vi "LDA_Align_PN_8 point.vi"(1 "Align Probe Using":enum16{"Green Beams", "Blue Beams"}(ring), 2 "Use Specification Beam Half-Angle":bool) -> (0 "Beam Data":T2={"Vg1 (Green 1 dir. vect.)"=[0.059117350659853476, -0.996541267827751, 0.05840068807144843], "Vg2  (Green 2 dir. vect.)"=[-0.05232536310393669, -0.9971561380468801, -0.054237373935992664], "Vb1 (Blue 1 dir. vect.)"=[-0.052923229613528855, -0.9969242065933935, 0.057803616456121795], "Vb2 (Blue 1 dir. vect.)"=[0.05971521716944564, -0.9967731992812374, -0.05364030232066602], "Porb (Orb XYZ posn. forced coplanar)"=[2201.0738225655555, -1199.3737231995547, 269.758310600838], "Porb (Orb XYZ posn. - allow skew)"=[2200.796256301178, -1199.3740953152687, 270.0329332816893], "Orb posn. uncertainty, +/- dx, dy, dz"=[0.13878313218879157, 0.00018605785703584843, 0.13731134042564008], "Vp (Actual Probe dir. vect)"=[0.003406702197773746, -0.9999920168246164, 0.0020882210543692924], "Yaw (deg)"=89.80480953887573, "Pitch (deg)"=0.11964634006213794, "In-Plane Roll (deg)"=45.305328966424156, "Beam Half Angle (deg)"=4.544091484248422, "B1 Close P11"=[0.0, 0.0, 0.0], "B1 Far P12"=[2158.01, -491.04, 229.28], "B2 Close P22"=[2158.01, -491.04, 229.28], "B2 Far P21"=[2158.01, -491.04, 229.28], "Projected Roll (deg)"=0.0, "Green Velocity Vector"=[0.0, 0.0, 0.0], "Blue Velocity Vector"=[0.0, 0.0, 0.0], "Probe is facing...."="-", "Calculation Method"=""} {"Vp (Actual Probe dir. vect)" format="%#_6f"; "Vg2  (Green 2 dir. vect.)" format="%#_6f"; "Vg1 (Green 1 dir. vect.)" format="%#_6f"})   [LabVIEW 2018]
uses:
  Controls/LDA_Beam_Cluster.ctl
  Gen Trav/Route mapping/Axis.ctl
  Controls/Tunnel_Coordinates.ctl
  Controls/Post_Process.ctl
  Controls/Setup.ctl
  Controls/User_Specific_mode.ctl
  Globals/LDA_meas_global_1.vi
  Globals/Trav_pos_global.vi
panel:
  out "8 Peaked positions":dbl[][](array[numeric])
  out "Peakup up inputs":dbl[][](array[numeric])
  out "Fixed Axis":T1
  out "png folder":path
  out "Taught point names":string[](array[string])
  out "Taught Positions":dbl[][](array[numeric])
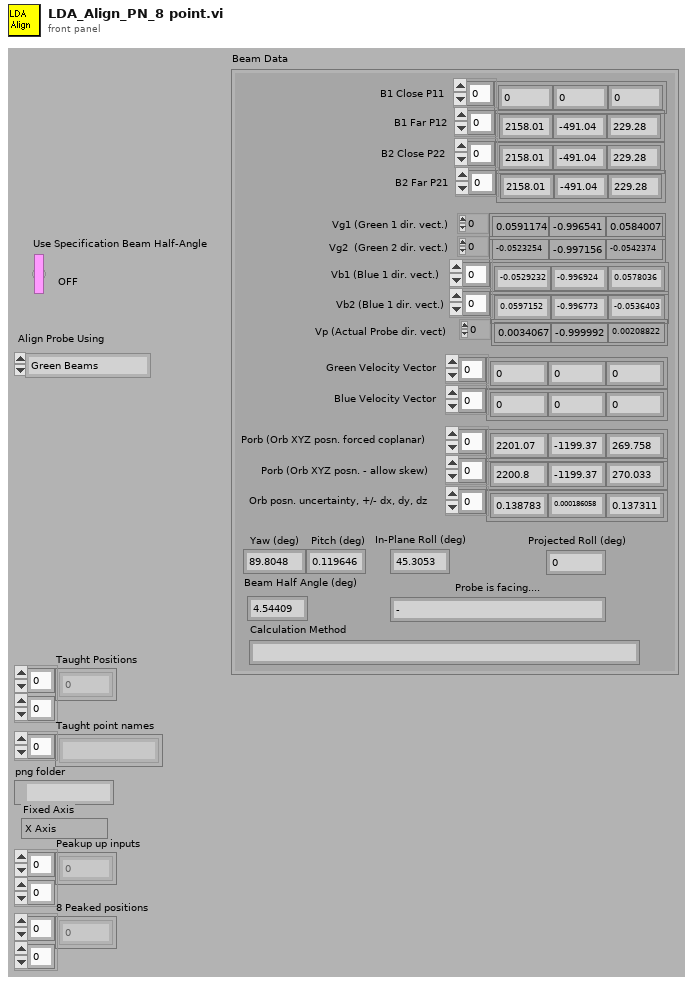
[diagram p1: front panel]
types:
  T1 = typedef "Axis.ctl" = enum16{"X Axis", "X Axis -ve", "Y Axis", "Y Axis -ve", "Z Axis", "Z Axis -ve"}
  T2 = typedef "LDA_Beam_Cluster.ctl" = cluster{"Vg1 (Green 1 dir. vect.)":dbl[], "Vg2  (Green 2 dir. vect.)":dbl[], "Vb1 (Blue 1 dir. vect.)":dbl[], "Vb2 (Blue 1 dir. vect.)":dbl[], "Porb (Orb XYZ posn. forced coplanar)":dbl[], "Porb (Orb XYZ posn. - allow skew)":dbl[], "Orb posn. uncertainty, +/- dx, dy, dz":dbl[], "Vp (Actual Probe dir. vect)":dbl[], "Yaw (deg)":dbl, "Pitch (deg)":dbl, "In-Plane Roll (deg)":dbl, "Beam Half Angle (deg)":dbl, "B1 Close P11":dbl[], "B1 Far P12":dbl[], "B2 Close P22":dbl[], "B2 Far P21":dbl[], "Projected Roll (deg)":dbl, "Green Velocity Vector":dbl[], "Blue Velocity Vector":dbl[], "Probe is facing....":string, "Calculation Method":string}
  T3 = typedef "Tunnel_Coordinates.ctl" = enum16{"Work in Tunnel Coordinates", "Work in Model Coordinates"}
  T4 = typedef "Setup.ctl" = enum16{"Run Program", "Show Setup", "Save Current Setup", "Setup Front Panel"}
  T5 = typedef "Post_Process.ctl" = enum16{"Take New Data", "Post Process Raw Data File"}
  T6 = typedef "User_Specific_mode.ctl" = enum16{"Check VI only", "Run VI"}
  T7 = enum16{"Load setup from excel file", "Save setup to excel file"}
  T8 = cluster{"second":i32, "minute":i32, "hour":i32, "day of month":i32, "month":i32, "year":i32, "day of week":i32, "day of year":i32, "is DST":i32}
  T9 = typedef "Multi_Run_Status.ctl" = enum16{"Continue", "Continue with Error", "Jump to Next Point", "Jump to Next Row", "Jump To Fall Back", "Terminate Run"}
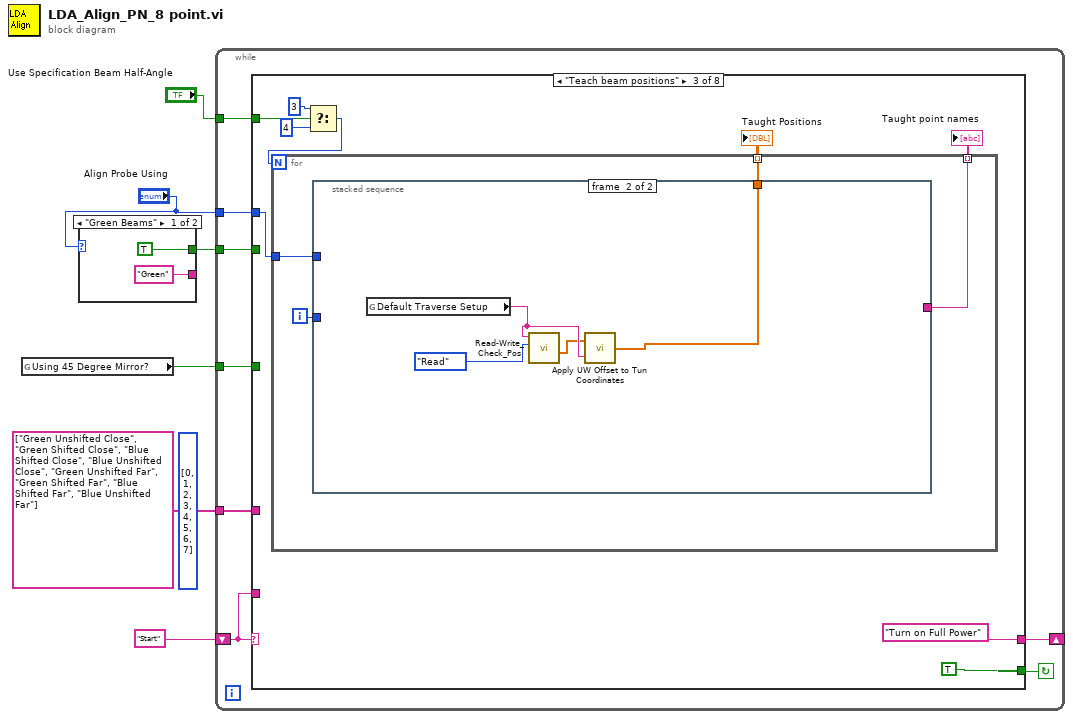
[diagram p0: block diagram]
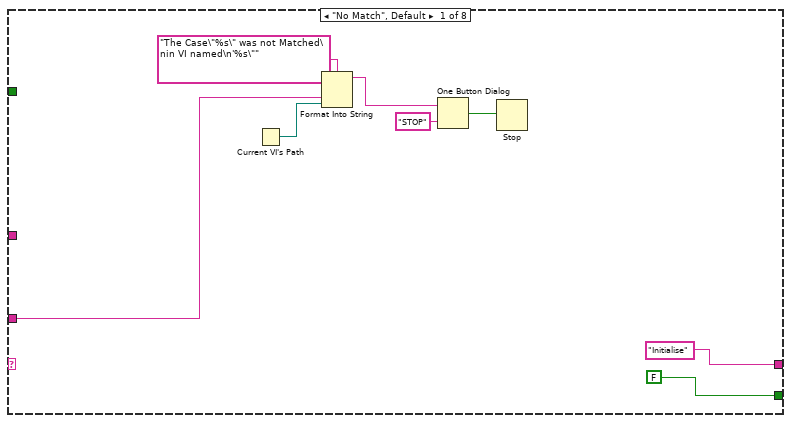
[diagram p2: hidden frame]
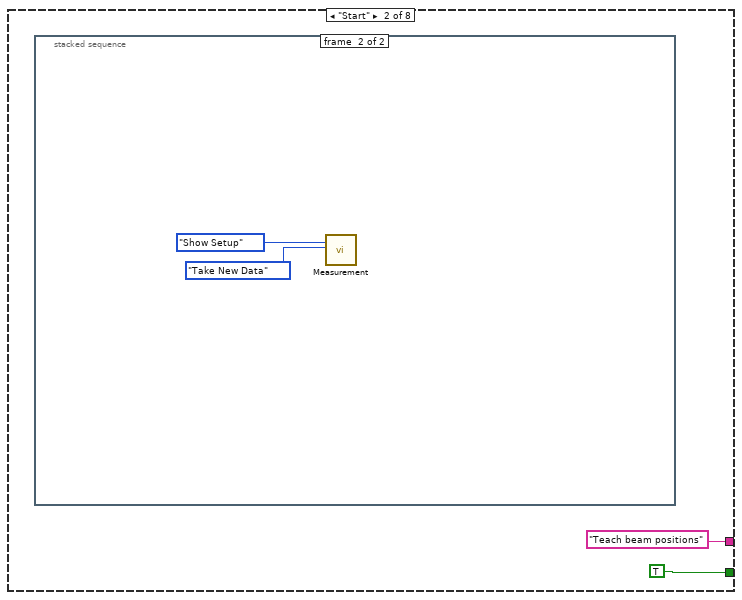
[diagram p3: hidden frame]
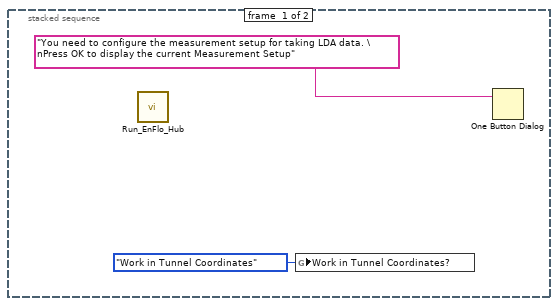
[diagram p4: hidden frame]
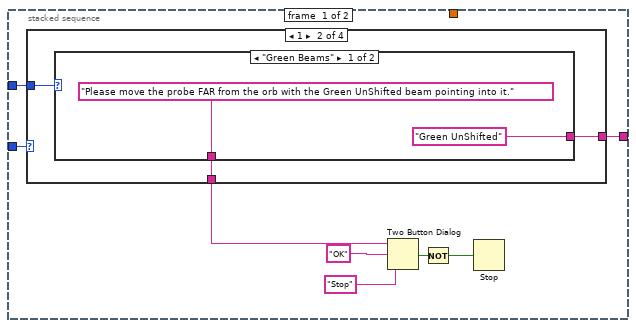
[diagram p5: hidden frame]
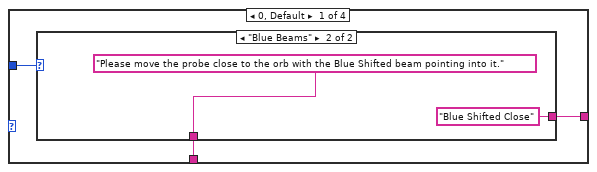
[diagram p6: hidden frame]
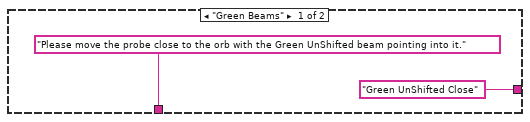
[diagram p7: hidden frame]
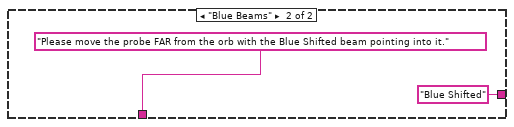
[diagram p8: hidden frame]
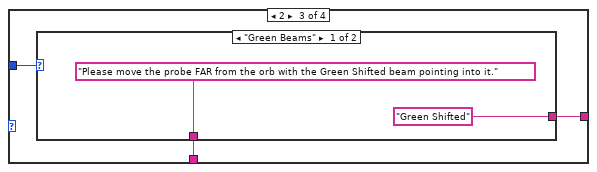
[diagram p9: hidden frame]
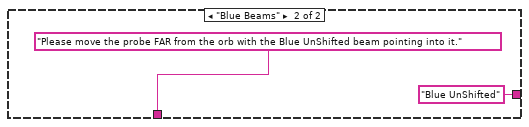
[diagram p10: hidden frame]
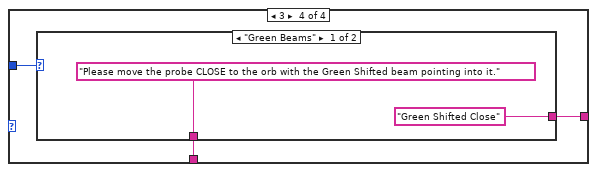
[diagram p11: hidden frame]
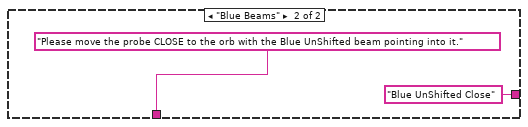
[diagram p12: hidden frame]
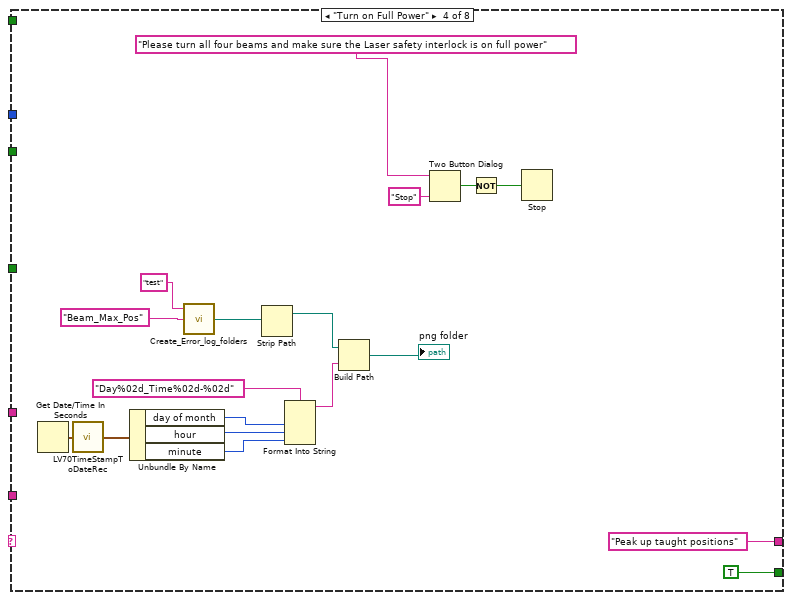
[diagram p13: hidden frame]
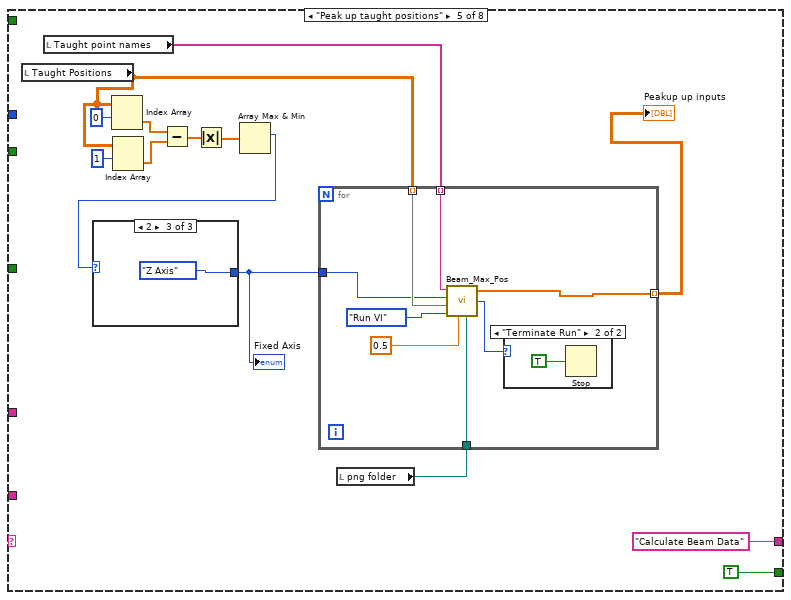
[diagram p14: hidden frame]
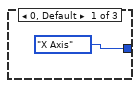
[diagram p15: hidden frame]
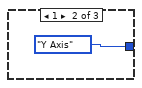
[diagram p16: hidden frame]
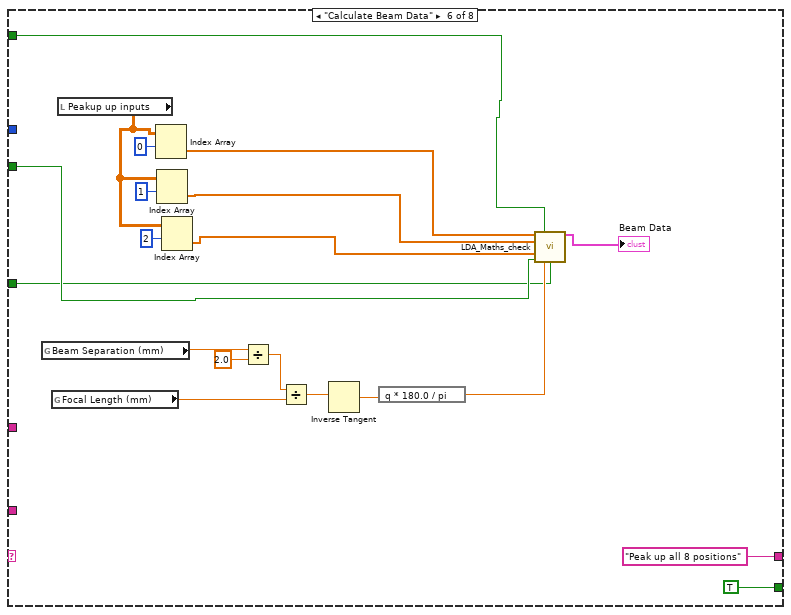
[diagram p18: hidden frame]
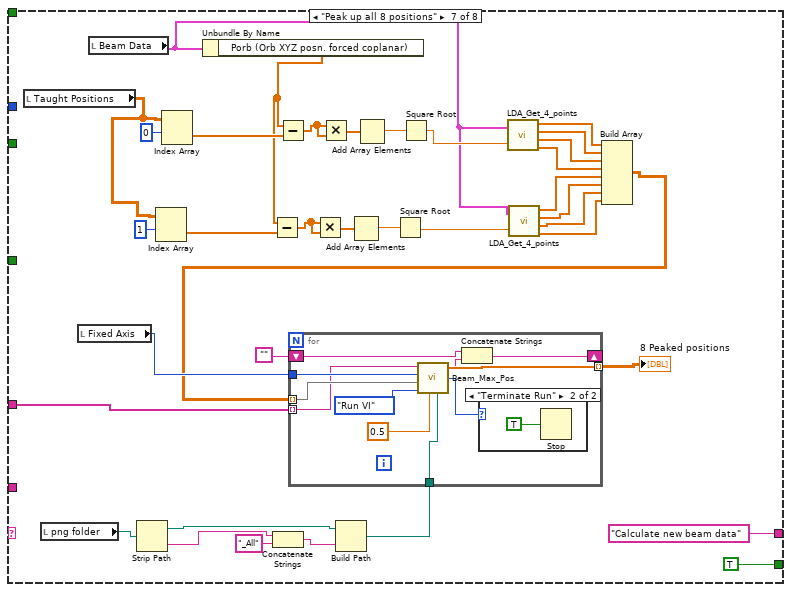
[diagram p19: hidden frame]
diagram:
  (unwired) i32[] [0, 1, 2, 3, 4, 5, 6, 7] ("appended array")
  n1 = global read "LDA_meas_global_1.vi" "Using 45 Degree Mirror?"() -> (w1:bool)
  n2 = case shown="\"Green Beams\"" "Align Probe Using" {
    tunnel: [TRUE FALSE] -> w3
    tunnel: ["Green" "Blue"] -> _
    frame "Green Beams" {
    }
    frame "Blue Beams" {
    }
  }
  n3 = while {
    shift-left: "Start" -> [w16]
    shift-right: [w17] -> _
    tunnel: "Align Probe Using" -> [w15]
    tunnel: "Use Specification Beam Half-Angle" -> [w14]
    tunnel: w3 -> [w13]
    tunnel: string[] ["Green Unshifted Close", "Green Shifted Close", "Blue Shifted Close", "Blue Unshifted Close", "Green Unshifted Far", "Green Shifted Far", "Blue Shifted Far", "Blue Unshifted Far"] ("appended array") -> [w12]
    tunnel: w1 -> [w11]
    stop <- w18 continue-if-true
    n4 = case shown="\"Teach beam positions\"" w16 {
      tunnel: [FALSE TRUE TRUE TRUE TRUE TRUE TRUE FALSE] -> w18
      tunnel: ["Initialise" "Teach beam positions" "Turn on Full Power" "Peak up taught positions" "Calculate Beam Data" "Peak up all 8 positions" "Calculate new beam data" "Log Check Angles panel"] -> w17
      tunnel: w16 -> [w21 _ _ _ _ _ _ _]
      tunnel: w15 -> [_ _ w39 _ _ _ _ _]
      tunnel: w14 -> [_ _ w36 _ _ w147 _ _]
      tunnel: w13 -> [_ _ _ _ _ w146 _ _]
      tunnel: w12 -> [_ _ _ _ _ _ w152 _]
      tunnel: w11 -> [_ _ _ _ _ w130 _ w198]
      frame "No Match", Default {
        n5 = Current VI's Path() -> (path=w20:path)
        n6 = Format Into String(format string="The Case\"%s\" was not Matched\nin VI named\n'%s\"" ("Format String"), w21, w20) -> (resulting string=w24:string)  [unwired: 2 in, 1 out]
        n7 = One Button Dialog(message=w24, button name ("OK")="STOP") -> (true=w22:bool)
        n8 = Stop(stop? (T)=w22) -> ()
      }
      frame "Start" {
        n9 = stacked-sequence {
          frame #0 {
            n10 = call "Run_EnFlo_Hub.vi"() -> ()  [unwired: 1 in, 7 out]
            n11 = global write "Trav_pos_global.vi" "Work in Tunnel Coordinates?"(Tunnel_Coordinates."Work in Tunnel Coordinates" ("Work in Tunnel Coordinates?")) -> ()
            n12 = One Button Dialog(message="You need to configure the measurement setup for taking LDA data. \nPress OK to display the current Measurement Setup") -> ()  [unwired: 1 in, 1 out]
          }
          frame #1 {
            n13 = call "Measurement.vi"("setup"=Setup."Show Setup", "Post Process"=Post_Process."Take New Data") -> ()  [unwired: 16 in, 2 out]
          }
        }
      }
      frame "Teach beam positions" {
        n14 = Select(t=3, s=w36, f=4) -> (s? t:f=w35:i32)
        n15 = for {
          N: w35 -> [_]
          tunnel: [w45] -> w34 mode=indexing
          tunnel: w39 -> [w44]
          tunnel: [w43] -> w33 mode=indexing
          i -> [w42]
          n16 = stacked-sequence {
            tunnel: [_ w82] -> w45
            tunnel: w44 -> [w52 _]
            tunnel: [w47 _] -> w43
            tunnel: w42 -> [w46 _]
            frame #0 {
              n17 = case shown="1" w46 {
                tunnel: [w56 w63 w70 w77] -> w53
                tunnel: w52 -> [w55 w62 w69 w76]
                tunnel: [w54 w61 w68 w75] -> w47
                frame 0, Default {
                  n18 = case shown="\"Blue Beams\"" w55 {
                    tunnel: ["Please move the probe close to the orb with the Green UnShifted beam pointing into it." ("message") "Please move the probe close to the orb with the Blue Shifted beam pointing into it." ("message")] -> w56
                    tunnel: ["Green UnShifted Close" "Blue Shifted Close"] -> w54
                    frame "Green Beams" {
                    }
                    frame "Blue Beams" {
                    }
                  }
                }
                frame 1 {
                  n19 = case shown="\"Green Beams\"" w62 {
                    tunnel: ["Please move the probe FAR from the orb with the Green UnShifted beam pointing into it." ("message") "Please move the probe FAR from the orb with the Blue Shifted beam pointing into it." ("message")] -> w63
                    tunnel: ["Green UnShifted" "Blue Shifted"] -> w61
                    frame "Green Beams" {
                    }
                    frame "Blue Beams" {
                    }
                  }
                }
                frame 2 {
                  n20 = case shown="\"Green Beams\"" w69 {
                    tunnel: ["Please move the probe FAR from the orb with the Green Shifted beam pointing into it." ("message") "Please move the probe FAR from the orb with the Blue UnShifted beam pointing into it." ("message")] -> w70
                    tunnel: ["Green Shifted" "Blue UnShifted"] -> w68
                    frame "Green Beams" {
                    }
                    frame "Blue Beams" {
                    }
                  }
                }
                frame 3 {
                  n21 = case shown="\"Green Beams\"" w76 {
                    tunnel: ["Please move the probe CLOSE to the orb with the Green Shifted beam pointing into it." ("message") "Please move the probe CLOSE to the orb with the Blue UnShifted beam pointing into it." ("message")] -> w77
                    tunnel: ["Green Shifted Close" "Blue UnShifted Close"] -> w75
                    frame "Green Beams" {
                    }
                    frame "Blue Beams" {
                    }
                  }
                }
              }
              n22 = Two Button Dialog(message=w53, 1:"Stop" ("F button name (\"Cancel\")"), 2:"OK" ("T button name (\"OK\")")) -> (T button?=w49:bool)
              n23 = Not(x=w49) -> (.not. x?=w48:bool)
              n24 = Stop(stop? (T)=w48) -> ()
            }
            frame #1 {
              n25 = global read "Trav_pos_global.vi" "Default Traverse Setup"() -> (w84:string)
              n26 = call "Read-Write_Check_Pos.vi"("Mode"=enum16{"Read", "Write"}."Read", "Traverse Name"=w84) -> ("Position Output"=w83:sgl[])  [unwired: 3 in, 2 out]
              n27 = call "Apply UW Offset to Tun Coordinates.vi"("Traverse Name"=w84, "Tunnel Coordinates"=w83) -> ("UW Offset Applied"=w82:sgl[])
            }
          }
        }
        "Taught Positions" <- w34
        "Taught point names" <- w33
      }
      frame "Turn on Full Power" {
        n28 = Get Date/Time In Seconds() -> (seconds since 1Jan1904=w86:timestamp)
        n29 = call <vilib>:"LV70TimeStampToDateRec.vi"("time stamp"=w86) -> ("date time rec"=w95:T8)
        n30 = Unbundle By Name(w95) -> ("day of month"=w92:i32, "hour"=w93:i32, "minute"=w94:i32)
        n31 = call "Create_Error_log_folders.vi"("Log Filename"="test", "Log Folder"="Beam_Max_Pos" ("name or relative path")) -> ("Server copy Location"=w87:path)  [unwired: 3 in, 2 out]
        n32 = Strip Path(path=w87) -> (stripped path=w96:path)  [unwired: 1 out]
        n33 = Format Into String(format string="Day%02d_Time%02d-%02d", w92, w93, w94) -> (resulting string=w97:string)  [unwired: 2 in, 1 out]
        n34 = Build Path(base path=w96, name or relative path=w97) -> (appended path=→"png folder":path)
        n35 = Two Button Dialog(message="Please turn all four beams and make sure the Laser safety interlock is on full power", 1:"Stop" ("F button name (\"Cancel\")")) -> (T button?=w101:bool)  [unwired: 1 out]
        n36 = Not(x=w101) -> (.not. x?=w102:bool)
        n37 = Stop(stop? (T)=w102) -> ()
      }
      frame "Peak up taught positions" {
        n38 = local read "Taught Positions"() -> (w108:dbl[][])
        n39 = local read "Taught point names"() -> (w107:string[])
        n40 = Index Array(array=w108, index (row)=0) -> (element=w111:dbl[])  [unwired: 1 in]
        n41 = Index Array(array=w108, index (row)=1) -> (element=w112:dbl[])  [unwired: 1 in]
        n42 = Subtract(x=w111, y=w112) -> (x-y=w113:dbl[])
        n43 = Absolute Value(x=w113) -> (abs(x)=w114:dbl[])
        n44 = Array Max & Min(array=w114) -> (max index (indices)=w115:i32)  [unwired: 3 out]
        n45 = case shown="2" w115 {
          tunnel: [Axis."X Axis" ("Fixed Axis") Axis."Y Axis" ("Fixed Axis") Axis."Z Axis" ("Fixed Axis")] -> w106
          frame 0, Default {
          }
          frame 1 {
          }
          frame 2 {
          }
        }
        "Fixed Axis" <- w106
        n46 = local read "png folder"() -> (w105:path)
        n47 = for {
          tunnel: w107 -> [w128] mode=indexing
          tunnel: w108 -> [w127] mode=indexing
          tunnel: w106 -> [w125]
          tunnel: w105 -> [w124]
          tunnel: [w123] -> w104 mode=indexing
          n48 = call "Beam_Max_Pos.vi"("Picture Log"=w124, "Search Step (mm)"=0.5, "Mode"=User_Specific_mode."Run VI", "Starting Position"=w127, "Fixed Axis"=w125, "Beam Name"=w128) -> ("Status"=w121:T9, "Beam maxima"=w123:dbl[])  [unwired: 1 in, 2 out]
          n49 = case shown="\"Terminate Run\"" w121 {
            frame "Continue", Default {
            }
            frame "Terminate Run" {
              n50 = Stop(stop? (T)=TRUE) -> ()
            }
          }
        }
        "Peakup up inputs" <- w104
      }
      frame "Calculate Beam Data" {
        n51 = global read "LDA_meas_global_1.vi" "Beam Separation (mm)"() -> (w133:dbl)
        n52 = global read "LDA_meas_global_1.vi" "Focal Length (mm)"() -> (w136:dbl)
        n53 = local read "Peakup up inputs"() -> (w139:dbl[][])
        n54 = Index Array(array=w139, index (row)=0) -> (element=w143:dbl[])  [unwired: 1 in]
        n55 = Index Array(array=w139, index (row)=1) -> (element=w144:dbl[])  [unwired: 1 in]
        n56 = Index Array(array=w139, index (row)=2) -> (element=w145:dbl[])  [unwired: 1 in]
        n57 = Divide(x=w133, y=2.0) -> (x/y=w135:dbl)
        n58 = Divide(x=w135, y=w136) -> (x/y=w138:dbl)
        n59 = Inverse Tangent(1:w138) -> (0:w137:dbl)
        n60 = expression code="q * 180.0 / pi"(w137) -> (w132:dbl)
        n61 = call "LDA_Maths_check.vi"("B1 Close P11"=w143, "Use Specification Beam Half-Angle"=w147, "B1 Far P12"=w144, "B2 Far P21"=w145, "Use Green Beams (True) or Blue Beams (False)"=w146, "Beam Half-Angle (deg)"=w132, "Using 45 Degree Mirror?"=w130) -> ("Beam Data"=→"Beam Data":T2)  [unwired: 8 out]
      }
      frame "Peak up all 8 positions" {
        n62 = local read "Taught Positions"() -> (w173:dbl[][])
        n63 = local read "png folder"() -> (w164:path)
        n64 = local read "Fixed Axis"() -> (w165:T1)
        n65 = local read "Beam Data"() -> (w171:T2)
        n66 = Strip Path(path=w164) -> (stripped path=w160:path, name=w163:string)
        n67 = Index Array(array=w173, index (row)=1) -> (element=w174:dbl[])  [unwired: 1 in]
        n68 = Index Array(array=w173, index (row)=0) -> (element=w183:dbl[])  [unwired: 1 in]
        n69 = Unbundle By Name(w171) -> ("Porb (Orb XYZ posn. forced coplanar)"=w151:dbl[])
        n70 = Subtract(x=w151, y=w174) -> (x-y=w178:dbl[])
        n71 = Concatenate Strings(w163, "_All" ("string")) -> (w161:string)
        n72 = Subtract(x=w151, y=w183) -> (x-y=w179:dbl[])
        n73 = Multiply(x=w178, y=w178) -> (x*y=w177:dbl[])
        n74 = Multiply(x=w179, y=w179) -> (x*y=w180:dbl[])
        n75 = Build Path(base path=w160, name or relative path=w161) -> (appended path=w150:path)
        n76 = Add Array Elements(numeric array=w177) -> (sum=w176:dbl)
        n77 = Add Array Elements(numeric array=w180) -> (sum=w181:dbl)
        n78 = Square Root(x=w176) -> (sqrt(x)=w170:dbl)
        n79 = Square Root(x=w181) -> (sqrt(x)=w172:dbl)
        n80 = call "LDA_Get_4_points.vi"("Beam Data"=w171, "L, Probe-Normal Distance"=w172) -> ("Pg1"=w169:dbl[], "Pg2"=w168:dbl[], "Pb1"=w167:dbl[], "Pb2"=w166:dbl[])
        n81 = call "LDA_Get_4_points.vi"("Beam Data"=w171, "L, Probe-Normal Distance"=w170) -> ("Pg1"=w157:dbl[], "Pg2"=w156:dbl[], "Pb1"=w158:dbl[], "Pb2"=w159:dbl[])
        n82 = Build Array(w169, w168, w167, w166, w157, w156, w158, w159) -> (w155:dbl[][])
        n83 = for {
          tunnel: w150 -> [w195]
          tunnel: [w194] -> w153 mode=indexing
          shift-right: [w191] -> _
          shift-left: "" -> [w193]
          tunnel: w155 -> [w188] mode=indexing
          tunnel: w165 -> [w187]
          tunnel: w152 -> [w186] mode=indexing
          n84 = call "Beam_Max_Pos.vi"("Picture Log"=w195, "Search Step (mm)"=0.5, "Mode"=User_Specific_mode."Run VI", "Starting Position"=w188, "Fixed Axis"=w187, "Beam Name"=w186) -> ("Status"=w189:T9, "Beam maxima"=w194:dbl[], "Message"=w192:string)  [unwired: 1 in, 1 out]
          n85 = Concatenate Strings(w193, w192) -> (w191:string)
          n86 = case shown="\"Terminate Run\"" w189 {
            frame "Continue", Default {
            }
            frame "Terminate Run" {
              n87 = Stop(stop? (T)=TRUE) -> ()
            }
          }
        }
        "8 Peaked positions" <- w153
      }
      frame "Calculate new beam data" {
        w211 = FALSE  # Use Green Beams (True) or Blue Beams (False)
        w228 = TRUE  # Use Green Beams (True) or Blue Beams (False)
        n88 = local read "8 Peaked positions"() -> (w209:dbl[][])
        n89 = Index Array(array=w209, index (row)=7) -> (element=w219:dbl[])  [unwired: 1 in]
        n90 = Index Array(array=w209, index (row)=3) -> (element=w218:dbl[])  [unwired: 1 in]
        n91 = Index Array(array=w209, index (row)=5) -> (element=w220:dbl[])  [unwired: 1 in]
        n92 = Index Array(array=w209, index (row)=6) -> (element=w217:dbl[])  [unwired: 1 in]
        n93 = Index Array(array=w209, index (row)=1) -> (element=w221:dbl[])  [unwired: 1 in]
        n94 = Index Array(array=w209, index (row)=4) -> (element=w222:dbl[])  [unwired: 1 in]
        n95 = Index Array(array=w209, index (row)=2) -> (element=w213:dbl[])  [unwired: 1 in]
        n96 = Index Array(array=w209, index (row)=0) -> (element=w226:dbl[])  [unwired: 1 in]
        n97 = call "LDA_Maths_check.vi"("B1 Close P11"=w213, "Use Specification Beam Half-Angle"=FALSE, "B1 Far P12"=w217, "B2 Close P22"=w218, "B2 Far P21"=w219, "Use Green Beams (True) or Blue Beams (False)"=w211, "Using 45 Degree Mirror?"=w198) -> ("Beam Data"=w199:T2)  [unwired: 1 in, 7 out]
        n98 = call "LDA_Maths_check.vi"("B1 Close P11"=w226, "Use Specification Beam Half-Angle"=FALSE, "B1 Far P12"=w222, "B2 Close P22"=w221, "B2 Far P21"=w220, "Use Green Beams (True) or Blue Beams (False)"=w228, "Using 45 Degree Mirror?"=w198) -> ("Beam Data"=w202:T2)  [unwired: 1 in, 7 out]
        n99 = Unbundle By Name(w202) -> ("Vg1 (Green 1 dir. vect.)"=w208:dbl[], "Vg2  (Green 2 dir. vect.)"=w207:dbl[])
        n100 = Unbundle By Name(w199) -> ("Vb1 (Blue 1 dir. vect.)"=w206:dbl[], "Vb2 (Blue 1 dir. vect.)"=w205:dbl[])
        n101 = call "Read_Write_Beam_Data.vi"("Beam Data In"=w199, "Mode"=T7."Save setup to excel file") -> ()  [unwired: 1 out]
        n102 = call "Read_Write_Beam_Data.vi"("Beam Data In"=w202, "Mode"=T7."Save setup to excel file") -> ()  [unwired: 1 out]
        n103 = call "LDA_Angle_Checks.vi"("Vg1"=w208, "Vg2"=w207, "Vb1"=w206, "Vb2"=w205) -> ()  [unwired: 16 out]
      }
    }
  }
